vi "TestInfo.vi"(7 "Set (f)":bool, 11 "PluginIniFilePaths":path[](array[path])) -> (3 "PluginIniFilePaths":path[](array[path]))   [LabVIEW 2014, in "WfrmModule.lvlib"]
uses:
  WfrmModule.lvlib
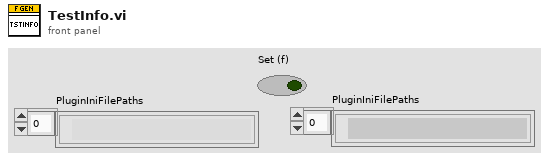
[diagram p1: front panel]
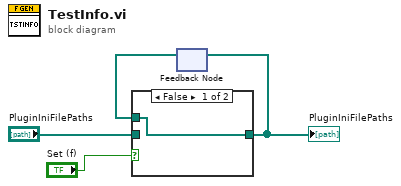
[diagram p0: block diagram]
diagram:
  n1 = feedback #1() -> (w3:path[])  [unwired: 1 in]
  n2 = case shown="False" "Set (f)" {
    tunnel: "PluginIniFilePaths" -> [_ w6]
    tunnel: [w5 w6] -> w1
    tunnel: w3 -> [w5 _]
    frame False {
    }
    frame True {
    }
  }
  "PluginIniFilePaths" <- w1
  n3 = feedback-in #1(w1) -> ()
